vi "Read Compatible Hardware Types.vi"(8 "error in (no error)":errorcluster, 11 "Strain in":refnum<class "Strain.lvclass">) -> (0 "error out":errorcluster, 2 "Compatible Hardware Types":string[](array[string]), 3 "Strain out":refnum<class "Strain.lvclass">)   [LabVIEW 2013, in "Strain.lvlib" / "Strain.lvclass"]
uses:
  Strain.lvclass
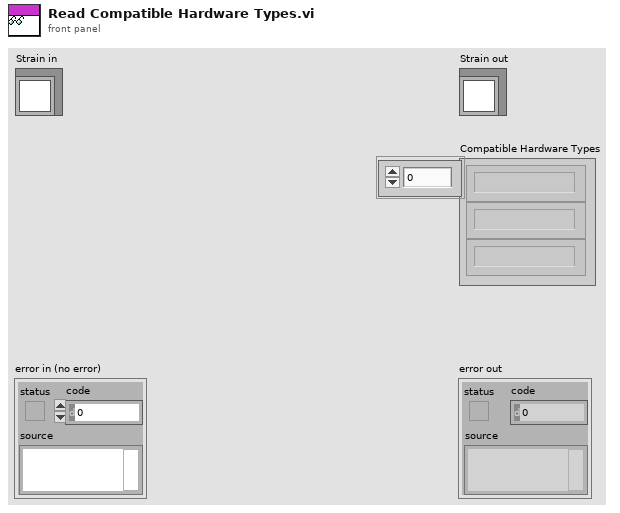
[diagram p1: front panel]
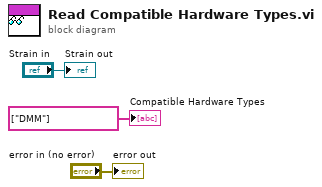
[diagram p0: block diagram]
diagram:
  "error out" <- "error in (no error)"
  "Strain out" <- "Strain in"
  "Compatible Hardware Types" <- string[] ["DMM"] ("Compatible Hardware Types")
